vi "Stop Handler Impl.vi"(8 "error in":errorcluster, 9 "stop button ref":refnum<vi>, 10 "stop server user event":T1, 11 "stop server broadcast event":refnum<user-event>) -> (0 "error out":errorcluster)   [LabVIEW 2021, in "NI Measurement Plug-In SDK.lvlib" / "IMeasurement Service.lvclass"]
uses:
  IMeasurement Service.lvclass
  Helpers/TypeDefs/Stop Server User Event.ctl
  NI Measurement Plug-In SDK.lvlib
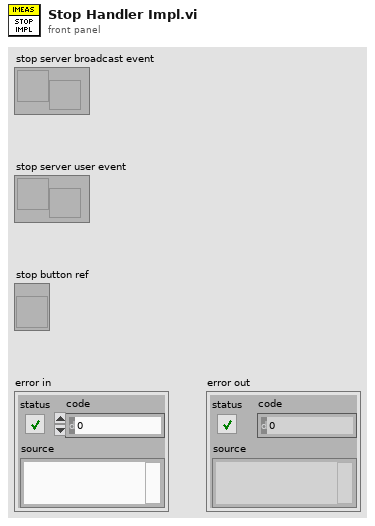
[diagram p1: front panel]
types:
  T1 = typedef "NI Measurement Plug-In SDK.lvlib/Stop Server User Event.ctl" = refnum<user-event>
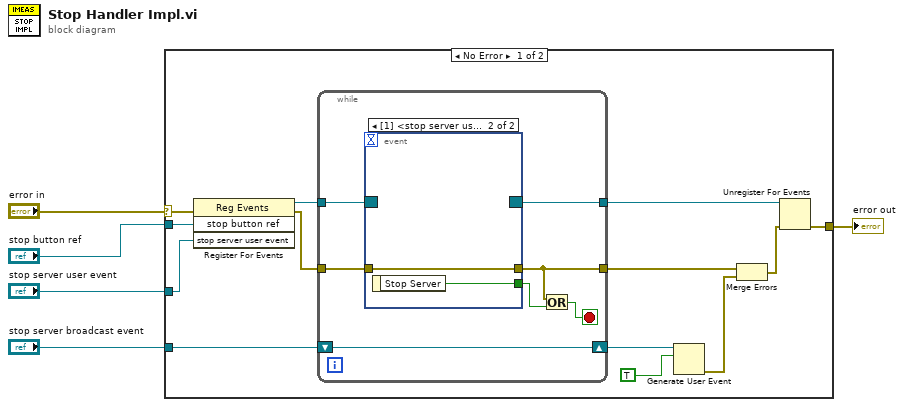
[diagram p0: block diagram]
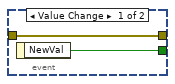
[diagram p2: hidden frame]
diagram:
  n1 = case shown="No Error" "error in" {
    selector: "error in" -> [w14 w30]
    tunnel: "stop server broadcast event" -> [w7 _]
    tunnel: "stop button ref" -> [w18 _]
    tunnel: [w17 w30] -> w3
    tunnel: "stop server user event" -> [w12 _]
    frame No Error {
      n2 = register-events(error in=w14, w18, w12) -> (reference out=w16:refnum<event-registration>, error out=w13:errorcluster)  [unwired: 1 in]
      n3 = while {
        tunnel: w16 -> [w25]
        tunnel: [w24] -> w15
        tunnel: [w21] -> w8
        tunnel: w13 -> [w23]
        shift-right: [w19] -> w6
        shift-left: w7 -> [w19]
        stop <- w20 stop-if-true
        n4 = event shown="[1] <stop server user event>: User Event" {
          selector: w25 -> [_ _]
          dyn-events: [_ _] -> w24
          timeout: _ -> [_ _]
          tunnel: [w26 w29] -> w22
          tunnel: [w27 w28] -> w21
          tunnel: w23 -> [w27 w28]
          event Value Change {
            n5 = event-data() -> ("NewVal"=w26:bool)  [unwired: 1 in]
          }
          event User Event {
            n6 = event-data() -> ("Stop Server"=w29:bool)  [unwired: 1 in]
          }
        }
        n7 = Or(x=w21, y=w22) -> (x .or. y?=w20:bool)
      }
      n8 = Generate User Event(user event=w6, event data cluster=TRUE ("event data")) -> (error out=w11:errorcluster)  [unwired: 2 in, 1 out]
      n9 = Merge Errors(w8, w11) -> (w10:errorcluster)
      n10 = Unregister For Events(event registration refnum=w15, error in=w10) -> (error out=w17:errorcluster)
    }
    frame Error {
    }
  }
  "error out" <- w3
